vi "Array Generator.vi"() -> ()   [LabVIEW 2024]
uses:
  <vilib>/Analysis/1siggen.llb/Ramp Pattern by Samples.vi
  <vilib>/Analysis/NI_AALBase.lvlib
panel:
  out "Array 3":dbl[](array[numeric])
  out "Array 2":dbl[](array[numeric])
  out "Ramp Pattern 2":dbl[](array[numeric])
  out "Array":dbl[](array[numeric])
  out "Ramp Pattern":dbl[](array[numeric])
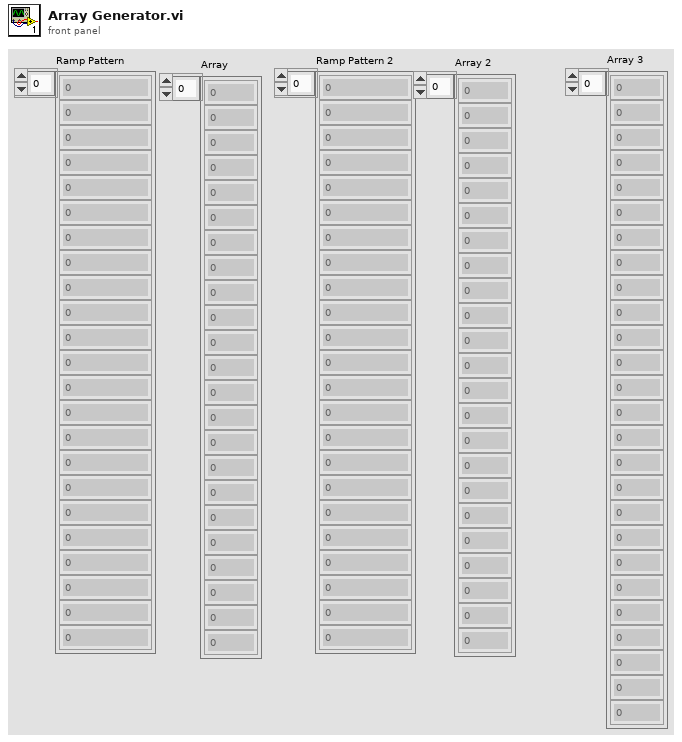
[diagram p1: front panel]
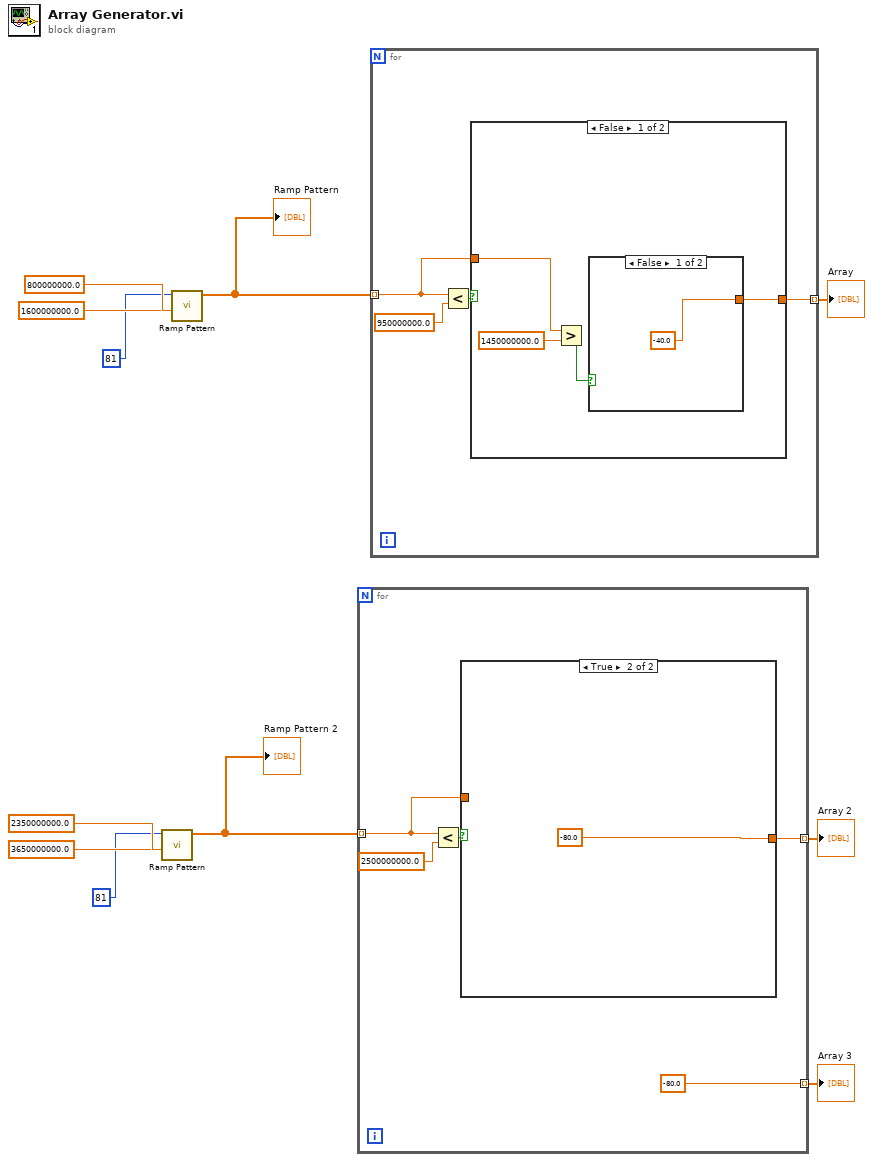
[diagram p0: block diagram]
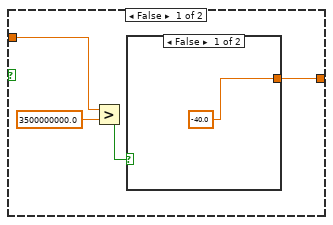
[diagram p2: hidden frame]
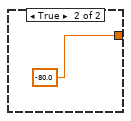
[diagram p3: hidden frame]
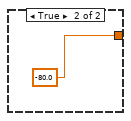
[diagram p4: hidden frame]
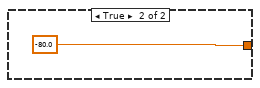
[diagram p5: hidden frame]
diagram:
  n1 = call-poly <vilib>:"Ramp Pattern.vi"("start"=2350000000.0, "end"=3650000000.0, "samples"=81) -> ("Ramp Pattern"=w3:dbl[])  [unwired: 7 in, 1 out]
  "Ramp Pattern 2" <- w3
  n2 = call-poly <vilib>:"Ramp Pattern.vi"("start"=800000000.0, "end"=1600000000.0, "samples"=81) -> ("Ramp Pattern"=w8:dbl[])  [unwired: 7 in, 1 out]
  "Ramp Pattern" <- w8
  n3 = for {
    tunnel: w3 -> [w14] mode=indexing
    tunnel: [w13] -> w2 mode=indexing
    tunnel: [-80.0 ("y")] -> w1 mode=indexing
    n4 = Less?(x=w14, y=2500000000.0) -> (x < y?=w15:bool)
    n5 = case shown="True" w15 {
      tunnel: w14 -> [w19 _]
      tunnel: [w17 -80.0 ("y")] -> w13
      frame False {
        n6 = Greater?(x=w19, y=3500000000.0) -> (0:w18:bool)
        n7 = case shown="False" w18 {
          tunnel: [-40.0 ("y") -80.0 ("y")] -> w17
          frame False {
          }
          frame True {
          }
        }
      }
      frame True {
      }
    }
  }
  "Array 2" <- w2
  "Array 3" <- w1
  n8 = for {
    tunnel: w8 -> [w25] mode=indexing
    tunnel: [w24] -> w7 mode=indexing
    n9 = Less?(x=w25, y=950000000.0) -> (x < y?=w26:bool)
    n10 = case shown="False" w26 {
      tunnel: w25 -> [w30 _]
      tunnel: [w28 -80.0 ("y")] -> w24
      frame False {
        n11 = Greater?(x=w30, y=1450000000.0) -> (0:w29:bool)
        n12 = case shown="False" w29 {
          tunnel: [-40.0 ("y") -80.0 ("y")] -> w28
          frame False {
          }
          frame True {
          }
        }
      }
      frame True {
      }
    }
  }
  "Array" <- w7
